vi "DELTA DIRAC.vi"() -> ()   [LabVIEW 2014]
uses:
  <vilib>/Analysis/2dsp.llb/Real FFT.vi
  <vilib>/Analysis/NI_AALPro.lvlib
  <vilib>/Analysis/NI_AALBase.lvlib
panel:
  out "error":i32
  out "Waveform Graph 2":dbl[](graph)
  in  "FFT size 2":i32=-1
  in  "shift?":bool
  out "Waveform Graph":dbl[](graph)
  in  "stop":bool
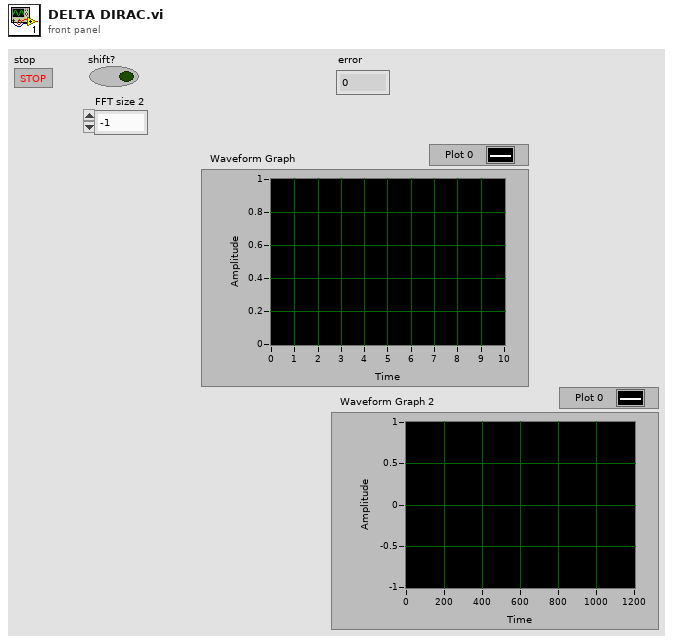
[diagram p1: front panel]
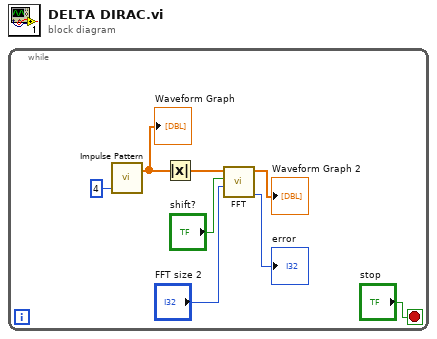
[diagram p0: block diagram]
diagram:
  n1 = while {
    stop <- "stop" stop-if-true
    n2 = call <vilib>:"Impulse Pattern.vi"("delay"=4) -> ("Impulse Pattern"=w7:dbl[])  [unwired: 2 in, 1 out]
    "Waveform Graph" <- w7
    n3 = Absolute Value(x=w7) -> (abs(x)=w6:dbl[])
    n4 = call-poly <vilib>:"FFT.vi"("FFT size"="FFT size 2", "shift?"="shift?", "X"=w6) -> ("error"=→"error":i32, "FFT {X}"=→"Waveform Graph 2":cdb[])  [unwired: 7 in]
  }
